vi "Delete Connection DVR.vi"(8 "error in (no error)":errorcluster, 11 "Connection DVR in":refnum<data-value>) -> (0 "error out":errorcluster, 3 "Connection out":refnum<class "Connection.lvclass">)   [LabVIEW 2012, in "MDSplus.lvlib" / "Connection.lvclass"]
uses:
  <vilib>/MDSplus/Classes/Connection_Class/Connection.lvclass
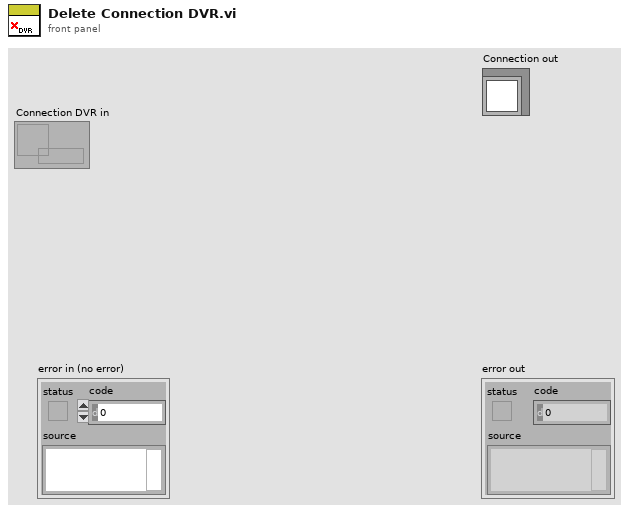
[diagram p1: front panel]
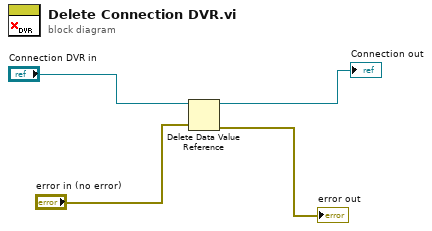
[diagram p0: block diagram]
diagram:
  n1 = Delete Data Value Reference(data value reference="Connection DVR in", error in="error in (no error)") -> (data value=→"Connection out":refnum<class "Connection.lvclass">, error out=→"error out":errorcluster)
